vi "Add Message to Bus Controller.vi"(4 "create timestamp channel":bool, 5 "create status channel for Rx and Tx":bool, 6 "parameters":T3(array[cluster]), 7 "number of words":u16, 8 "error in":errorcluster, 9 "direction":T4, 10 "name":string, 11 "port in":T1 format="%.0x") -> (0 "error out":errorcluster, 2 "message":T1=18446744073709551615 format="%.0x", 3 "port out":T1 format="%.0x")   [LabVIEW 2020, in "Ballard MIL-STD-1553 Scripting.lvlib"]
uses:
  Ballard MIL-STD-1553 Scripting.lvlib
  Shared/Direction.ctl
  Shared/Parameter Definition.ctl
  <vilib>/NI VeriStand/Custom Device API/Custom Device Item Ref.ctl
  Constants.vi
  <vilib>/NI VeriStand/Custom Device API/Custom Device API.lvlib
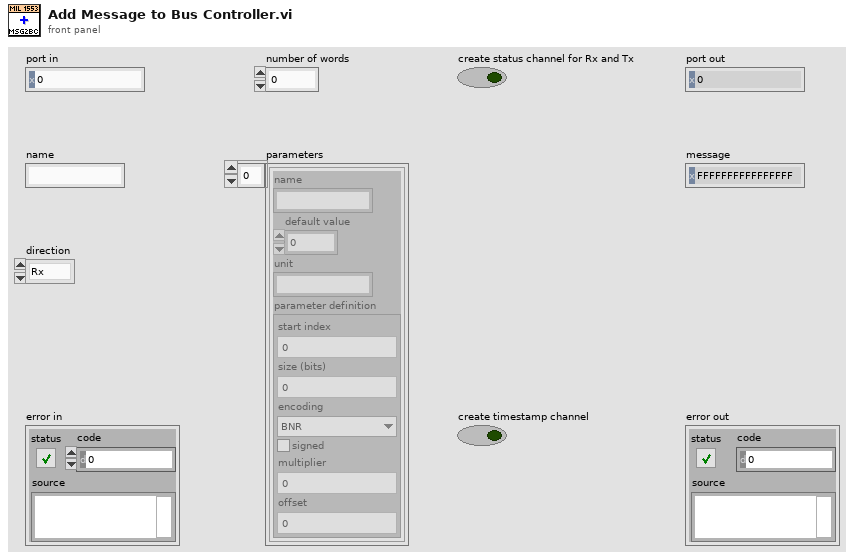
[diagram p1: front panel]
types:
  T1 = typedef "Custom Device API.lvlib/Custom Device Item Ref.ctl" = u64
  T2 = typedef "Parameter Definition.ctl" = cluster{"start index":i32, "size (bits)":i32, "encoding":enum16{"BNR", "BCD", "Discrete"}, "signed":bool, "multiplier":dbl, "offset":dbl}
  T3 = cluster{"name":string, "default value":dbl, "unit":string, "parameter definition":T2}[]
  T4 = typedef "Direction.ctl" = enum16{"Rx", "Tx"}
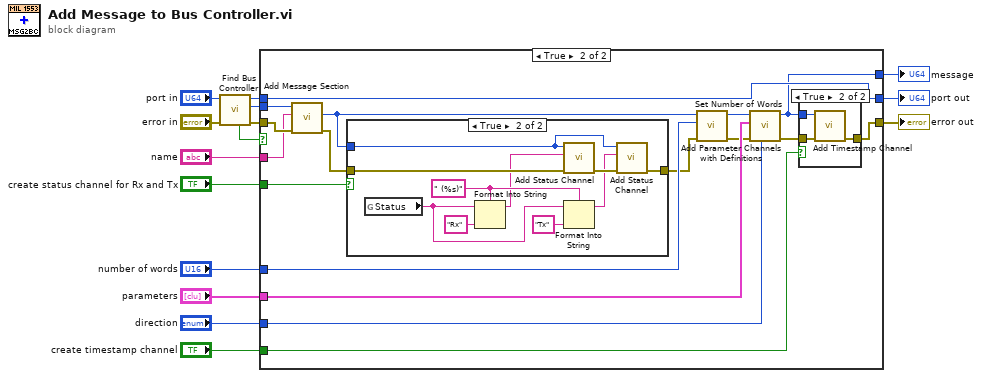
[diagram p0: block diagram]
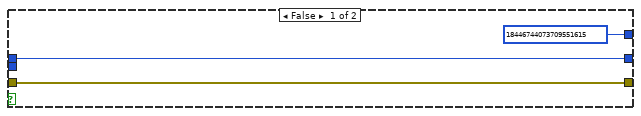
[diagram p2: hidden frame]
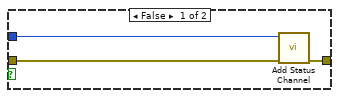
[diagram p3: hidden frame]
diagram:
  n1 = call "Find Bus Controller.vi"("error in"="error in", "port in"="port in") -> ("error out"=w7:errorcluster, "bus controller"=w6:T1, "port out"=w5:T1, "found?"=w4:bool)  [unwired: 6 in]
  n2 = case shown="True" w4 {
    tunnel: w5 -> [w18 w26]
    tunnel: w6 -> [_ w34]
    tunnel: w7 -> [w17 w35]
    tunnel: [w17 w24] -> w8
    tunnel: [w18 w26] -> w9
    tunnel: "number of words" -> [_ w33]
    tunnel: "parameters" -> [_ w32]
    tunnel: "name" -> [_ w29]
    tunnel: "direction" -> [_ w28]
    tunnel: "create timestamp channel" -> [_ w27]
    tunnel: "create status channel for Rx and Tx" -> [_ w21]
    tunnel: [T1 18446744073709551615 ("message out") w19] -> w1
    frame False {
    }
    frame True {
      n3 = call "Add Message Section.vi"("error in"=w35, "message name"=w29, "bus controller in"=w34) -> ("error out"=w23:errorcluster, "message"=w22:T1)  [unwired: 6 in, 1 out]
      n4 = case shown="True" w21 {
        tunnel: w23 -> [w38 w48]
        tunnel: w22 -> [w36 w39]
        tunnel: [w37 w40] -> w20
        frame False {
          n5 = call "Add Status Channel.vi"("error in"=w38, "section reference"=w36) -> ("error out"=w37:errorcluster)  [unwired: 8 in, 1 out]
        }
        frame True {
          w44 = " (%s)" ("format string")
          n6 = global read "Constants.vi" "Status"() -> (w43:string)
          n7 = Format Into String(format string=w44, initial string=w43, "Rx" ("Status")) -> (resulting string=w42:string)  [unwired: 1 in, 1 out]
          n8 = call "Add Status Channel.vi"("error in"=w48, "name (empty = \"Status\")"=w42, "section reference"=w39) -> ("error out"=w47:errorcluster)  [unwired: 7 in, 1 out]
          n9 = Format Into String(format string=w44, initial string=w43, "Tx" ("Status")) -> (resulting string=w41:string)  [unwired: 1 in, 1 out]
          n10 = call "Add Status Channel.vi"("error in"=w47, "name (empty = \"Status\")"=w41, "section reference"=w39) -> ("error out"=w40:errorcluster)  [unwired: 7 in, 1 out]
        }
      }
      n11 = call "Set Number of Words.vi"("error in"=w20, "number of words"=w33, "message in"=w22) -> ("error out"=w30:errorcluster, "message out"=w31:T1)  [unwired: 7 in]
      n12 = call "Add Parameter Channels with Definitions.vi"("direction"=w28, "error in"=w30, "parameters"=w32, "message in"=w31) -> ("error out"=w25:errorcluster, "message out"=w19:T1)  [unwired: 6 in]
      n13 = case shown="True" w27 {
        tunnel: w25 -> [w49 w52]
        tunnel: w19 -> [_ w51]
        tunnel: [w49 w50] -> w24
        frame False {
        }
        frame True {
          n14 = call "Add Timestamp Channel.vi"("error in"=w52, "message section"=w51) -> ("error out"=w50:errorcluster)  [unwired: 8 in, 1 out]
        }
      }
    }
  }
  "port out" <- w9
  "error out" <- w8
  "message" <- w1
